vi "Save strain data.vi"(8 "Error In":errorcluster, 10 "Data":dbl[][](array[numeric])) -> (0 "Error Out":errorcluster, 3 "File name":path)   [LabVIEW 2015]
uses:
  File/Controls/File formats.ctl
  <vilib>/Utility/file.llb/Write Delimited Spreadsheet (DBL).vi
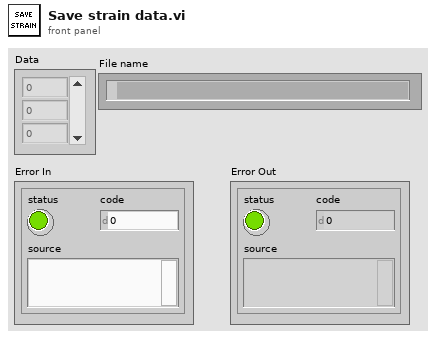
[diagram p1: front panel]
types:
  T1 = typedef "File formats.ctl" = enum16{"TDMS", "ASCII", "BINARY"}
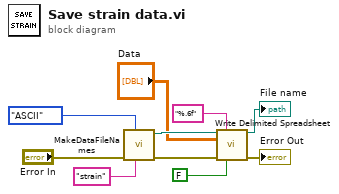
[diagram p0: block diagram]
diagram:
  n1 = call "MakeDataFileNames.vi"("File Prefix"="strain" ("File Name Prefix"), "File format"=File_formats."ASCII", "Error In"="Error In") -> ("Error Out"=w3:errorcluster, "Data File  Path"=w7:path)  [unwired: 5 in, 2 out]
  n2 = call-poly <vilib>:"Write Delimited Spreadsheet.vi"("file path (dialog if empty)"=w7, "format (%.3f)"="%.6f", "2D data"="Data", "error in (no error)"=w3, "transpose? (F)"=FALSE ("transpose? (no:F)")) -> ("new file path (Not A Path if cancelled)"=→"File name":path, "error out"=→"Error Out":errorcluster)  [unwired: 9 in]
